vi "消息推送.vi"(7 "枚举":enum16{"短信", "电话"}(ring), 8 "error in (no error)":errorcluster caption="错误输入（无错误）", 9 "分析":string="1、建议排查管路是否异常\n2、供电情况是否正常", 10 "内容":string="故障告警", 11 "站点":string="测试点") -> (0 "error out":errorcluster caption="错误输出")   [LabVIEW 2016, in "Alarm interface.lvlib" / "短信语音库.lvlib"]
uses:
  Alarm interface.lvlib
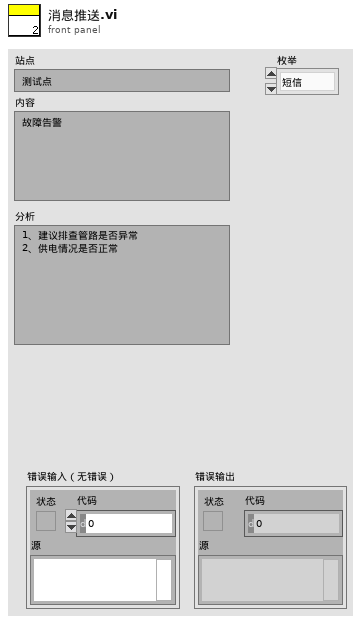
[diagram p1: front panel]
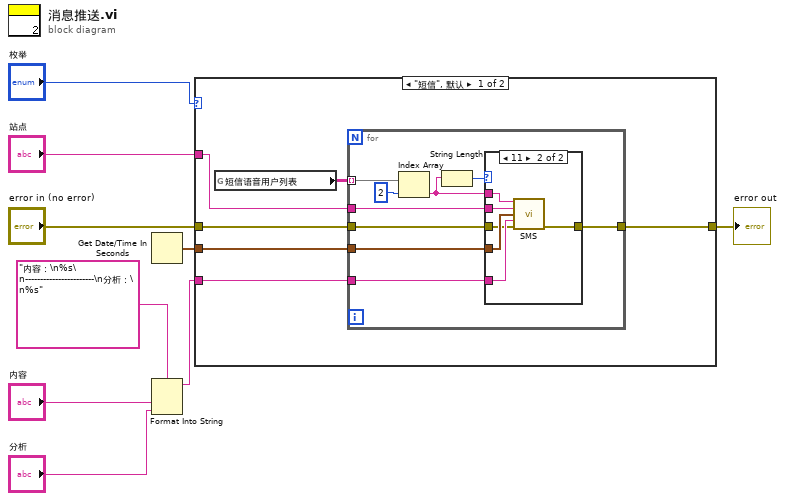
[diagram p0: block diagram]
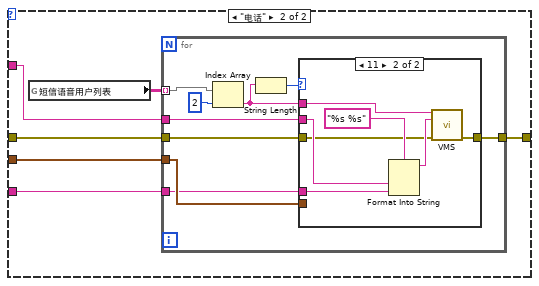
[diagram p3: hidden frame]
diagram:
  n1 = Get Date/Time In Seconds() -> (seconds since 1Jan1904=w6:timestamp)
  n2 = Format Into String(format string="内容：\n%s\n-----------------------\n分析：\n%s" ("格式字符串"), "内容", "分析") -> (resulting string=w1:string)  [unwired: 2 in, 1 out]
  n3 = case shown="\"短信\", 默认" "枚举" {
    tunnel: "站点" -> [w15 w37]
    tunnel: w6 -> [w14 w36]
    tunnel: w1 -> [w13 w35]
    tunnel: [w11 w34] -> w4
    tunnel: "error in (no error)" -> [w12 w33]
    frame "短信", Default {
      n4 = global read "断电保存全局.vi" "短信语音用户列表"() -> (w10:string[][])
      n5 = for {
        tunnel: w10 -> [w18] mode=indexing
        tunnel: w15 -> [w23]
        tunnel: w14 -> [w22]
        tunnel: w13 -> [w21]
        tunnel: w12 -> [w20]
        tunnel: [w19] -> w11
        n6 = Index Array(array=w18, index=2 ("索引")) -> (element=w16:string)
        n7 = String Length(string=w16) -> (length=w24:i32)
        n8 = case shown="11" w24 {
          tunnel: w16 -> [_ w31]
          tunnel: w23 -> [_ w30]
          tunnel: w22 -> [_ w29]
          tunnel: w21 -> [_ w28]
          tunnel: w20 -> [w25 w27]
          tunnel: [w25 w26] -> w19
          frame 0, Default {
          }
          frame 11 {
            n9 = call "SMS.vi"("PhoneNumbers"=w31, "站点"=w30, "时间标识"=w29, "内容"=w28, "error in (no error)"=w27) -> ("error out"=w26:errorcluster)  [unwired: 8 in, 2 out]
          }
        }
      }
    }
    frame "电话" {
      n10 = global read "断电保存全局.vi" "短信语音用户列表"() -> (w32:string[][])
      n11 = for {
        tunnel: w32 -> [w38] mode=indexing
        tunnel: w37 -> [w45]
        tunnel: w36 -> [w44]
        tunnel: w35 -> [w43]
        tunnel: [w42] -> w34
        tunnel: w33 -> [w41]
        n12 = Index Array(array=w38, index=2 ("索引")) -> (element=w39:string)
        n13 = String Length(string=w39) -> (length=w46:i32)
        n14 = case shown="11" w46 {
          tunnel: w39 -> [_ w50]
          tunnel: w45 -> [_ w52]
          tunnel: w44 -> [_ _]
          tunnel: w43 -> [_ w51]
          tunnel: [w47 w49] -> w42
          tunnel: w41 -> [w47 w48]
          frame 0, Default {
          }
          frame 11 {
            n15 = Format Into String(format string="%s %s" ("格式字符串"), w52, w51) -> (resulting string=w53:string)  [unwired: 2 in, 1 out]
            n16 = call "VMS.vi"("PhoneNumbers"=w50, "内容"=w53, "error in (no error)"=w48) -> ("error out"=w49:errorcluster)  [unwired: 10 in, 2 out]
          }
        }
      }
    }
  }
  "error out" <- w4
